vi "Actor Core.vi"(8 "error in":errorcluster, 11 "Nested in":refnum<class "Camera Worker.lvclass">) -> (0 "error out":errorcluster, 3 "Actor out":refnum<class "Actor.lvclass">)   [LabVIEW 2024, in "Camera Worker.lvlib" / "Camera Worker.lvclass"]
doc: "(<B>Filename</B>: Actor Framework.lvlib:Actor.lvclass:Actor Core.vi)\n\nReceives messages to the actor, reacts to them, and initiates any error handling that may shut the actor down.\n\nDescendant classes may override this VI to append parallel tasks for the actor to complete while it handles messages. Overrides use the Call Parent Method node."
uses:
  Camera Worker.lvclass
  <vilib>/ActorFramework/Actor/Actor.lvclass/Actor.ctl
  <vilib>/ActorFramework/Message Enqueuer/Message Enqueuer.lvclass/Message Enqueuer.ctl
  Camera Worker.lvclass/Camera Worker.ctl
  <vilib>/ActorFramework/Actor/Actor.lvclass
  <vilib>/ActorFramework/Actor Framework.lvlib
  Camera Worker Messages/Read Images Msg/Read Images Msg.lvclass
  C:/Program Files/National Instruments/LabVIEW 2025/vi.lib/ActorFramework/Actor/Actor.lvclass
  C:/Program Files/National Instruments/LabVIEW 2025/vi.lib/ActorFramework/Message/Message.lvclass
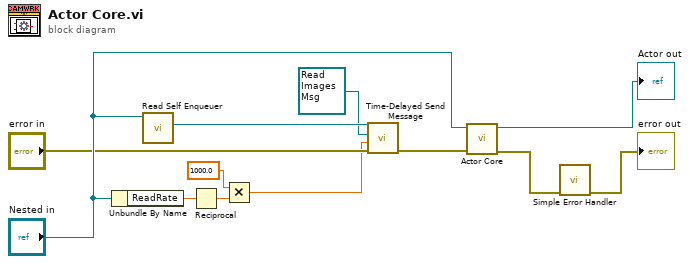
[diagram p0: block diagram]
diagram:
  n1 = Unbundle By Name("Nested in") -> ("ReadRate"=w10:dbl)
  n2 = call <vilib>:"Read Self Enqueuer.vi"("Actor"="Nested in") -> ("Self Enqueuer"=w6:refnum<class "Message Enqueuer.lvclass">)  [unwired: 10 in]
  n3 = Reciprocal(x=w10) -> (1/x=w9:dbl)
  n4 = Multiply(x=1000.0, y=w9) -> (x*y=w3:dbl)
  n5 = call <vilib>:"Time-Delayed Send Message.vi"("error in (no error)"="error in", "Milliseconds To Wait"=w3, "Message"=refnum<class "Read Images Msg.lvclass"> refnum ("Camera Worker.lvlib:Read Images Msg.lvclass"), "Message Enqueuer"=w6) -> ("error out"=w4:errorcluster)  [unwired: 6 in, 1 out]
  n6 = call-parent "Actor Core.vi"("error in"=w4, "Actor in"="Nested in") -> ("error out"=w12:errorcluster, "Actor out"=→"Actor out":refnum<class "Actor.lvclass">)  [unwired: 8 in]
  n7 = call <vilib>:"Simple Error Handler.vi"("error in (no error)"=w12) -> ("error out"=→"error out":errorcluster)  [unwired: 4 in, 4 out]
